vi "Day 3.vi"() -> ()   [LabVIEW 2020]
uses:
  Calculation Select_ENUM.ctl
  <vilib>/Utility/file.llb/Read Delimited Spreadsheet (string).vi
panel:
  out "Life Support Rating":u32
  out "Power Consumption":u32
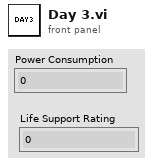
[diagram p1: front panel]
types:
  T1 = typedef "Calculation Select_ENUM.ctl" = enum16{"Oxy Gen Rating", "C02 Scrub Rating"}
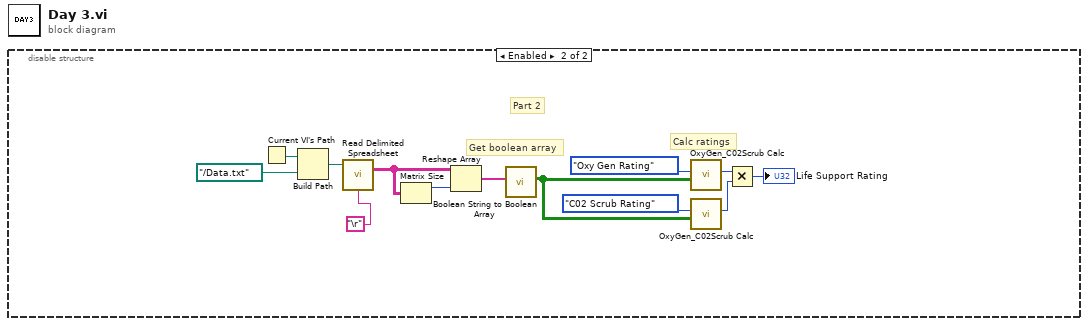
[diagram p0: block diagram]
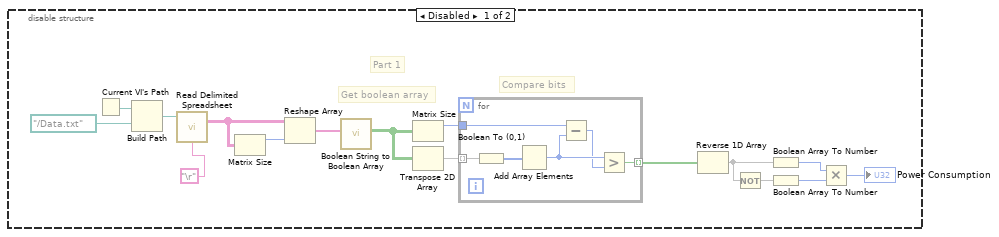
[diagram p2: hidden frame]
diagram:
  n1 = disable-structure shown="Enabled" {
    frame Disabled {
      # "Part 1"
      # "Compare bits"
      # "Get boolean array"
      n2 = Current VI's Path() -> (path=w15:path)
      n3 = Build Path(base path=w15, name or relative path=path "../Data.txt" ("file path (dialog if empty)")) -> (appended path=w13:path)
      n4 = call-poly <vilib>:"Read Delimited Spreadsheet.vi"("file path (dialog if empty)"=w13, "delimiter (\\t)"="\r") -> ("all rows"=w11:string[][])  [unwired: 8 in, 5 out]
      n5 = Matrix Size(0:w11) -> (1:w12:i32)  [unwired: 1 out]
      n6 = Reshape Array(w11, w12) -> (w2:string[])
      n7 = call "Boolean String to Boolean Array.vi"("Diagnostic Data"=w2) -> ("Diagostic Array Out"=w1:bool[][])  [unwired: 10 in]
      n8 = Matrix Size(0:w1) -> (1:w9:i32)  [unwired: 1 out]
      n9 = Transpose 2D Array(2D array=w1) -> (transposed array=w10:bool[][])
      n10 = for {
        tunnel: w10 -> [w22] mode=indexing
        tunnel: w9 -> [w20]
        tunnel: [w17] -> w8 mode=indexing
        n11 = Boolean To (0,1)(Boolean=w22) -> (0, 1=w21:i16[])
        n12 = Add Array Elements(numeric array=w21) -> (sum=w19:i16)
        n13 = Subtract(x=w20, y=w19) -> (x-y=w18:i32)
        n14 = Greater?(x=w19, y=w18) -> (0:w17:bool)
      }
      n15 = Reverse 1D Array(array=w8) -> (reversed array=w6:bool[])
      n16 = Not(x=w6) -> (.not. x?=w7:bool[])
      n17 = Boolean Array To Number(Boolean array=w6) -> (number=w5:u32)
      n18 = Boolean Array To Number(Boolean array=w7) -> (number=w4:u32)
      n19 = Multiply(x=w5, y=w4) -> (x*y=→"Power Consumption":u32)
    }
    frame Enabled {
      # "Part 2"
      # "Calc ratings"
      # "Get boolean array"
      n20 = Current VI's Path() -> (path=w34:path)
      n21 = Build Path(base path=w34, name or relative path=path "../Data.txt" ("file path (dialog if empty)")) -> (appended path=w32:path)
      n22 = call-poly <vilib>:"Read Delimited Spreadsheet.vi"("file path (dialog if empty)"=w32, "delimiter (\\t)"="\r") -> ("all rows"=w30:string[][])  [unwired: 8 in, 5 out]
      n23 = Matrix Size(0:w30) -> (1:w31:i32)  [unwired: 1 out]
      n24 = Reshape Array(w30, w31) -> (w26:string[])
      n25 = call "Boolean String to Boolean Array.vi"("Diagnostic Data"=w26) -> ("Diagostic Array Out"=w25:bool[][])  [unwired: 10 in]
      n26 = call "OxyGen_C02Scrub Calc.vi"("Diagnostic Data In"=w25, "Calculation Select"=Calculation_Select_ENUM."Oxy Gen Rating") -> ("Oxy Gen/C02 Scrub Rating Out"=w28:u32)  [unwired: 9 in]
      n27 = call "OxyGen_C02Scrub Calc.vi"("Diagnostic Data In"=w25, "Calculation Select"=Calculation_Select_ENUM."C02 Scrub Rating") -> ("Oxy Gen/C02 Scrub Rating Out"=w27:u32)  [unwired: 9 in]
      n28 = Multiply(x=w28, y=w27) -> (x*y=→"Life Support Rating":u32)
    }
  }
